vi "Globals.vi"(7 "Action":T1, 9 "Values in":string[](array[string]), 10 "Key":string) -> (1 "Values out":string[](array[string]), 2 "Found?":bool, 3 "Globals":map{string, string[]}(c390), 5 "Keys":string[](array[string]))   [LabVIEW 2021, in "HttpServer.lvlib"]
uses:
  HttpServer.lvlib
  TypeDefs/Action.ctl
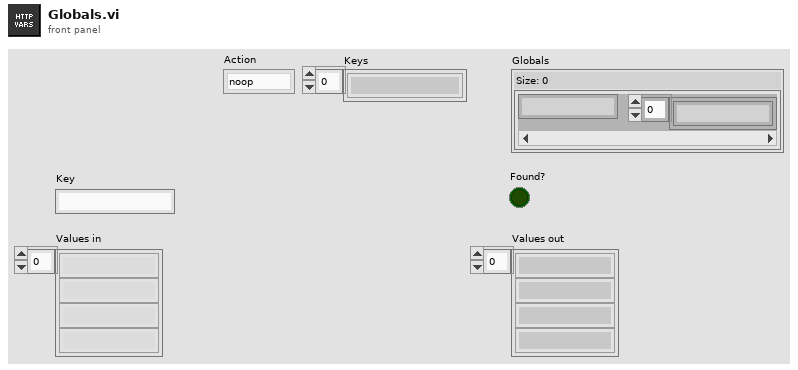
[diagram p1: front panel]
types:
  T1 = typedef "HttpServer.lvlib/Action.ctl" = enum8{"noop", "add", "get", "set", "remove"}
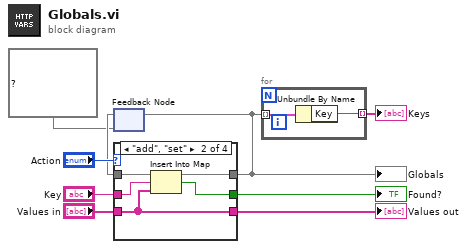
[diagram p0: block diagram]
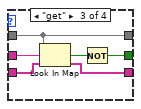
[diagram p3: hidden frame]
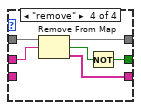
[diagram p4: hidden frame]
diagram:
  n1 = feedback #1(map{string, string[]} {} ("Keys")) -> (w8:map{string, string[]})
  n2 = case shown="\"add\", \"set\"" "Action" {
    tunnel: w8 -> [w10 w15 w21 w27]
    tunnel: [w10 w14 w21 w26] -> w5
    tunnel: "Key" -> [_ w13 w20 w25]
    tunnel: "Values in" -> [_ w11 w19 _]
    tunnel: [_ w11 w18 w24] -> w3
    tunnel: [_ w12 w16 w22] -> w2
    frame "noop" {
    }
    frame "add", "set" {
      n3 = Insert Into Map(map in=w15, key=w13, value=w11) -> (map out=w14:map{string, string[]}, key already included?=w12:bool)  [unwired: 1 out]
    }
    frame "get" {
      n4 = Look In Map(map=w21, key=w20, default value=w19) -> (key not found?=w17:bool, value=w18:string[])
      n5 = Not(x=w17) -> (.not. x?=w16:bool)
    }
    frame "remove" {
      n6 = Remove From Map(10:w25, 11:w27) -> (1:w24:string[], 2:w23:bool, 3:w26:map{string, string[]})
      n7 = Not(x=w23) -> (.not. x?=w22:bool)
    }
  }
  "Values out" <- w3
  "Found?" <- w2
  "Globals" <- w5
  n8 = feedback-in #1(w5) -> ()
  n9 = for {
    tunnel: w5 -> [w29] mode=indexing
    tunnel: [w28] -> w4 mode=indexing
    n10 = Unbundle By Name(w29) -> ("Key"=w28:string)
  }
  "Keys" <- w4
